vi "Open_Results_File_Excel.vi"(8 "error in (no error)":errorcluster, 11 "path to file":path) -> (0 "error out":errorcluster)   [LabVIEW 2018]
doc: "This VI Uses the ActiveX interface to search an Excel Worksheet and return the Column and Row for a specified value."
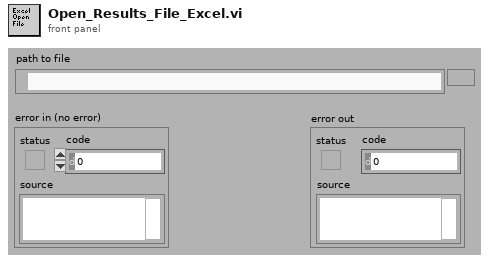
[diagram p1: front panel]
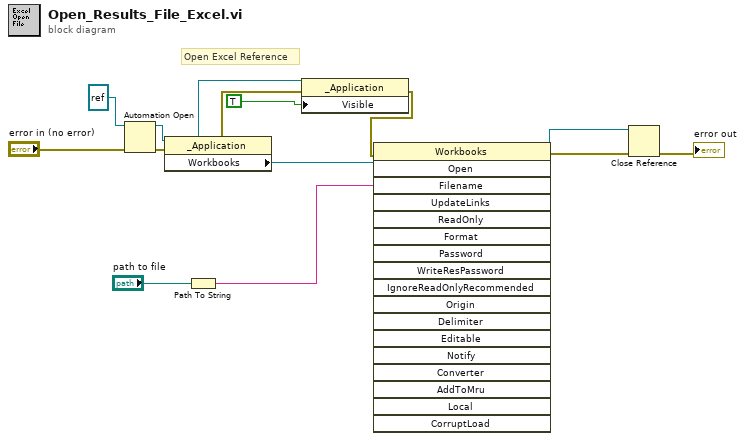
[diagram p0: block diagram]
diagram:
  # "Open Excel Reference"
  n1 = Automation Open(error in (no error)="error in (no error)", Automation Refnum=refnum<k7> refnum ("Excel._Application")) -> (Automation Refnum=w8:refnum<k7>, error out=w7:errorcluster)  [unwired: 2 out]
  n2 = property class="_Application"(reference=w8, error in=w7) -> (reference out=w6:refnum<k7>, error out=w4:errorcluster, "Workbooks"=w3:refnum<k7>)
  n3 = Path To String(path="path to file") -> (string=w9:string)
  n4 = property class="_Application"(reference=w6, error in=w4, "Visible"=TRUE) -> (error out=w2:errorcluster)  [unwired: 1 out]
  n5 = invoke class="Workbooks" method="Open"(reference=w3, error in=w2, "Filename"=w9) -> (reference out=w11:refnum<k7>, error out=w10:errorcluster)  [unwired: 15 in, 16 out]
  n6 = Close Reference(reference=w11, error in (no error)=w10) -> (error out=→"error out":errorcluster)
